vi "Pre Launch Init.vi"(11 "Spectroscopy_Controller in":refnum<class "Spectroscopy_Controller.lvclass">) -> (0 "error out":errorcluster, 3 "Spectroscopy_Controller out":refnum<class "Spectroscopy_Controller.lvclass">)   [LabVIEW 2023, in "Spectroscopy_Controller.lvlib" / "Spectroscopy_Controller.lvclass"]
doc: "(<B>Filename</B>: Actor Framework.lvlib:Actor.lvclass:Pre Launch Init.vi)\n\nDefines behavior that occurs after the Launch Nested Actor method is invoked but before the actor's Actor Core method begins running.\n\nBy default, this method does nothing. A descendant class may override it to define behavior."
uses:
  Spectroscopy_Controller.lvclass
  Spectroscopy_Controller.lvclass/Spectroscopy_Controller.ctl
  <vilib>/ActorFramework/Actor/Actor.lvclass
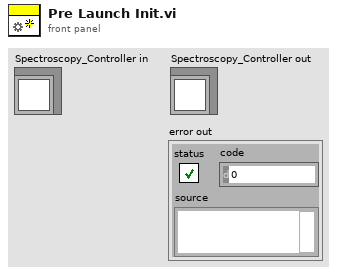
[diagram p1: front panel]
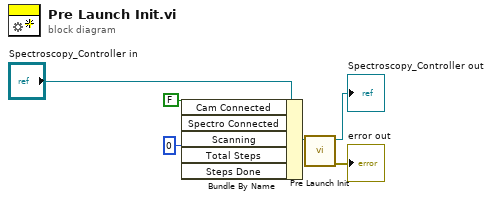
[diagram p0: block diagram]
diagram:
  w3 = u16 0 ("Total Steps")
  w4 = FALSE ("Cam Connected")
  n1 = Bundle By Name(cluster="Spectroscopy_Controller in", "Cam Connected"=w4, "Spectro Connected"=w4, "Scanning"=w4, "Total Steps"=w3, "Steps Done"=w3) -> (w1:refnum<class "Spectroscopy_Controller.lvclass">)
  n2 = call-parent "Pre Launch Init.vi"("Actor in"=w1) -> ("error out"=→"error out":errorcluster, "Actor out"=→"Spectroscopy_Controller out":refnum<class "Spectroscopy_Controller.lvclass">)  [unwired: 9 in]
